vi "模块启用配置框.vi"() -> ()   [LabVIEW 2016]
uses:
  <vilib>/Utility/config.llb/NI_LVConfig.lvlib
panel:
  in  "超标留样启用":bool
  in  "取消":bool
  in  "确认":bool
  in  "CODMn启用":bool caption="CODMn禁用"
  in  "质控单元启用":bool caption="质控单元禁用"
  in  "总磷总氮启用":bool caption="总磷总氮禁用"
  in  "流量计启用":bool caption="流量计禁用"
  in  "氨氮启用":bool caption="氨氮禁用"
  in  "多参数启用":bool caption="多参数禁用"
  in  "CODcr启用":bool caption="CODcr禁用"
  # "模块启用配置"
  # "说明:\n选择所需要启动的模块,并按确认,软件将重启生效."
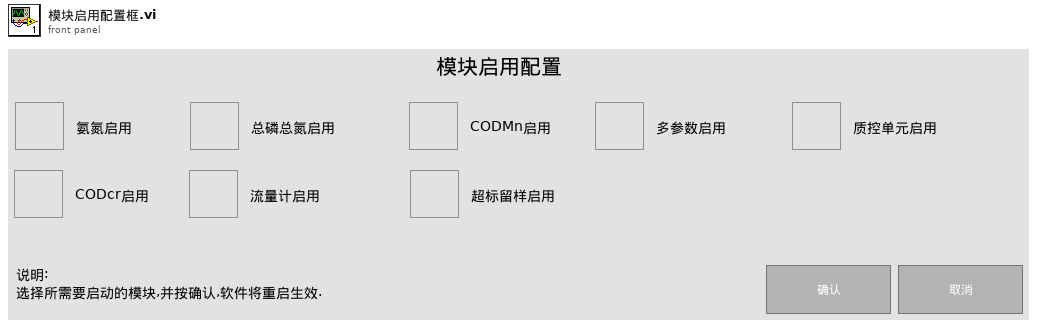
[diagram p1: front panel]
types:
  T1 = typedef "NI_LVConfig.lvlib/Config Data RefNum.ctl" = refnum<k1>
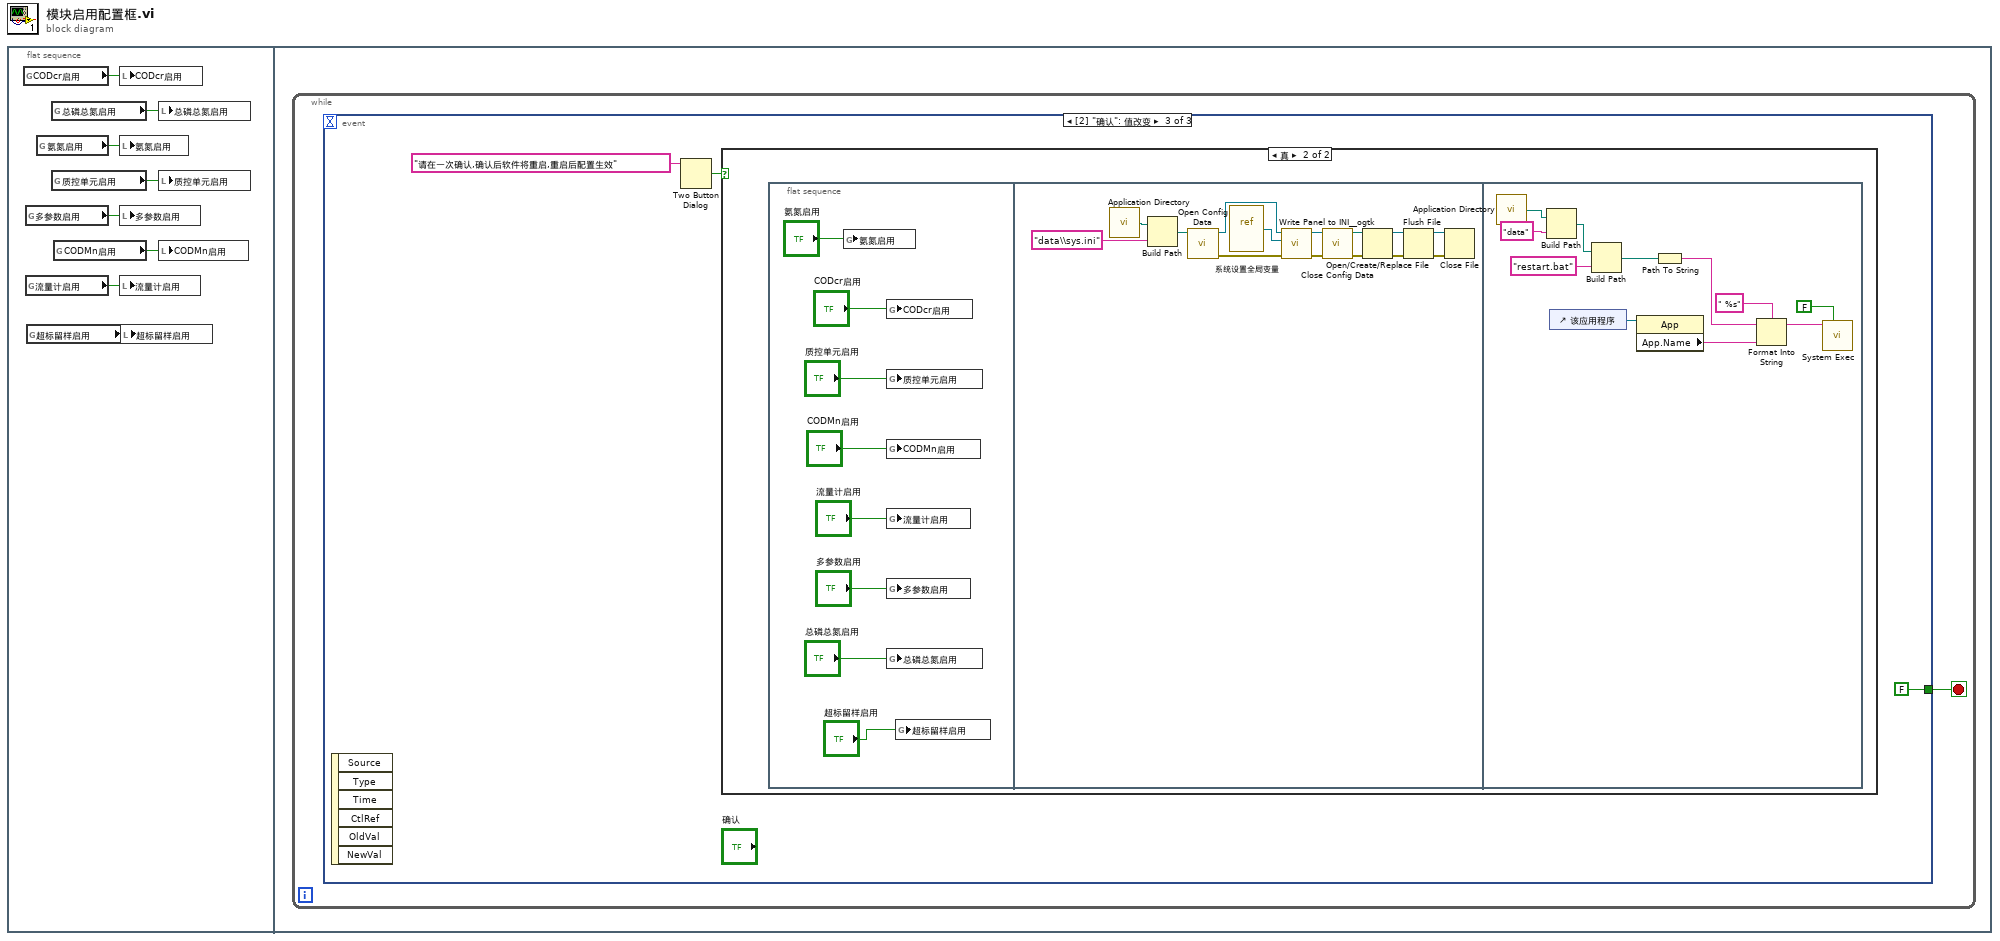
[diagram p0: block diagram]
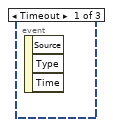
[diagram p2: hidden frame]
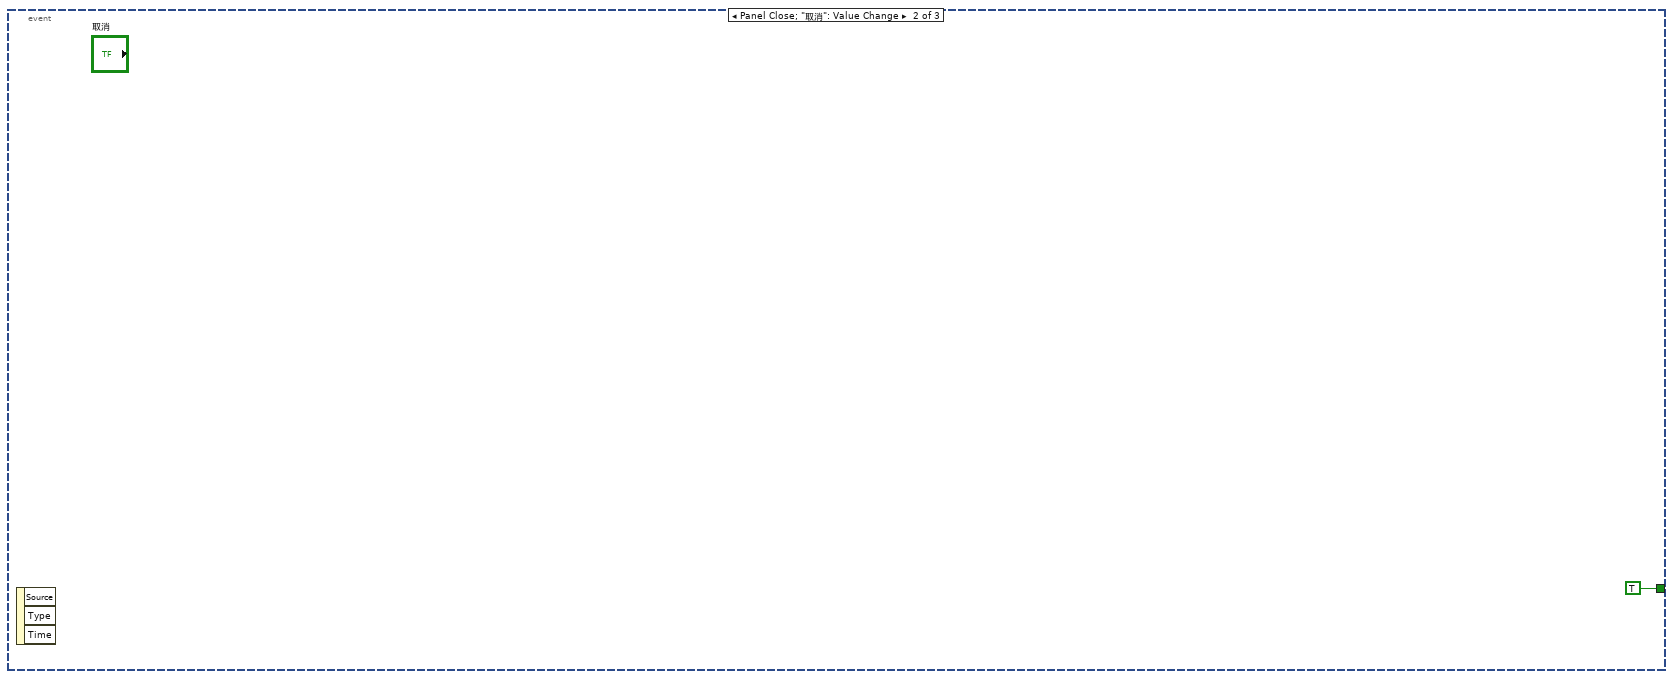
[diagram p3: hidden frame]
diagram:
  n1 = flat-sequence {
    frame #0 {
      n2 = global read "系统设置全局变量.vi" "CODcr启用"() -> (w8:bool)
      n3 = global read "系统设置全局变量.vi" "多参数启用"() -> (w6:bool)
      n4 = global read "系统设置全局变量.vi" "流量计启用"() -> (w5:bool)
      n5 = global read "系统设置全局变量.vi" "超标留样启用"() -> (w1:bool)
      n6 = global read "系统设置全局变量.vi" "氨氮启用"() -> (w4:bool)
      n7 = global read "系统设置全局变量.vi" "总磷总氮启用"() -> (w7:bool)
      n8 = global read "系统设置全局变量.vi" "质控单元启用"() -> (w2:bool)
      n9 = global read "系统设置全局变量.vi" "CODMn启用"() -> (w3:bool)
      n10 = local write "CODcr启用"(w8) -> ()
      n11 = local write "氨氮启用"(w4) -> ()
      n12 = local write "多参数启用"(w6) -> ()
      n13 = local write "流量计启用"(w5) -> ()
      n14 = local write "超标留样启用"(w1) -> ()
      n15 = local write "总磷总氮启用"(w7) -> ()
      n16 = local write "质控单元启用"(w2) -> ()
      n17 = local write "CODMn启用"(w3) -> ()
    }
    frame #1 {
      n18 = while {
        stop <- w9 stop-if-true
        n19 = event shown="[2] \"确认\": 值改变" {
          selector: _ -> [_ _ _]
          dyn-events: _ -> [_ _ _]
          timeout: _ -> [_ _ _]
          tunnel: [_ TRUE FALSE] -> w9
          event Timeout {
            n20 = event-data() -> ()  [unwired: 1 in, 3 out]
          }
          event Panel Close; "取消": Value Change {
            n21 = event-data() -> ()  [unwired: 1 in, 3 out]
          }
          event "确认": Value Change {
            n22 = event-data() -> ()  [unwired: 1 in, 6 out]
            n23 = Two Button Dialog(message="请在一次确认,确认后软件将重启,重启后配置生效" ("消息")) -> (T button?=w11:bool)  [unwired: 2 in]
            n24 = case shown="真" w11 {
              frame False {
              }
              frame True {
                n25 = flat-sequence {
                  frame #0 {
                    n26 = global write "系统设置全局变量.vi" "氨氮启用"("氨氮启用") -> ()
                    n27 = global write "系统设置全局变量.vi" "CODcr启用"("CODcr启用") -> ()
                    n28 = global write "系统设置全局变量.vi" "质控单元启用"("质控单元启用") -> ()
                    n29 = global write "系统设置全局变量.vi" "CODMn启用"("CODMn启用") -> ()
                    n30 = global write "系统设置全局变量.vi" "流量计启用"("流量计启用") -> ()
                    n31 = global write "系统设置全局变量.vi" "多参数启用"("多参数启用") -> ()
                    n32 = global write "系统设置全局变量.vi" "总磷总氮启用"("总磷总氮启用") -> ()
                    n33 = global write "系统设置全局变量.vi" "超标留样启用"("超标留样启用") -> ()
                  }
                  frame #1 {
                    n34 = call <vilib>:"Application Directory.vi"() -> ("Application Directory"=w35:path)
                    n35 = Build Path(base path=w35, name or relative path="data\\sys.ini" ("名称或相对路径")) -> (appended path=w33:path)
                    n36 = call <vilib>:"Open Config Data.vi"("configuration file path"=w33) -> ("error out"=w29:errorcluster, "refnum"=w32:T1)  [unwired: 8 in, 1 out]
                    n37 = vi-ref "系统设置全局变量.vi"() -> (w31:refnum<vi>)
                    n38 = call <userlib>:"Write Panel to INI__ogtk.vi"("error in (no error)"=w29, "VI ref"=w31, "refnum"=w32) -> ("error out"=w28:errorcluster, "refnum out"=w30:T1)  [unwired: 7 in]
                    n39 = call <vilib>:"Close Config Data.vi"("error in (no error)"=w28, "refnum"=w30) -> ("error out"=w23:errorcluster, "file path"=w22:path)  [unwired: 8 in]
                    n40 = Open/Create/Replace File(file path (use dialog)=w22, error in=w23) -> (refnum out=w26:refnum<file>, error out=w27:errorcluster)  [unwired: 4 in, 1 out]
                    n41 = Flush File(refnum=w26, error in=w27) -> (refnum out=w25:refnum<file>, error out=w24:errorcluster)
                    n42 = Close File(refnum=w25, error in=w24) -> ()  [unwired: 2 out]
                  }
                  frame #2 {
                    n43 = call <vilib>:"Application Directory.vi"() -> ("Application Directory"=w45:path)
                    n44 = Build Path(base path=w45, name or relative path="data" ("名称或相对路径")) -> (appended path=w43:path)
                    n45 = control-ref of="该应用程序"() -> (w46:refnum<vi>)
                    n46 = Build Path(base path=w43, name or relative path="restart.bat" ("名称或相对路径")) -> (appended path=w41:path)
                    n47 = property class="App"(reference=w46) -> ("App.Name"=w38:string)  [unwired: 1 in, 2 out]
                    n48 = Path To String(path=w41) -> (string=w40:string)
                    n49 = Format Into String(format string=" %s" ("格式字符串"), initial string=w40, w38) -> (resulting string=w37:string)  [unwired: 1 in, 1 out]
                    n50 = call <vilib>:"System Exec.vi"("wait until completion? (T)"=FALSE, "command line"=w37) -> ()  [unwired: 6 in, 4 out]
                  }
                }
              }
            }
          }
        }
      }
    }
  }
